vi "Run.vi"(8 "error in (no error)":errorcluster, 10 "OTP Cluster Out":T1, 11 "Measurements in":refnum<class "Measurement.lvclass">) -> (0 "error out":errorcluster, 1 "Parameters":cluster{"Name":string, "Value":string}[](array[cluster]), 2 "Canceled":bool, 3 "Measurements out":refnum<class "Measurement.lvclass">)   [LabVIEW 2020, in "Measurement.lvclass"]
doc: "This is the main test vi. It is here that the test is implemented."
uses:
  Measurement.lvclass
  Controls/OTP_Cluster.ctl
  Controls/Run States.ctl
  Devices/Controls/Change setting mode enum.ctl
  Measurement.lvclass/Measurement.ctl
  Support VI/Update parameters (array).vi
  Devices/Device.lvclass
  Devices/PIC-device/PIC-Device.lvclass
  Instruments/Power Supply/Power Supply.lvclass
  Instruments/Digital Multimeter/Digital Multimeter.lvclass
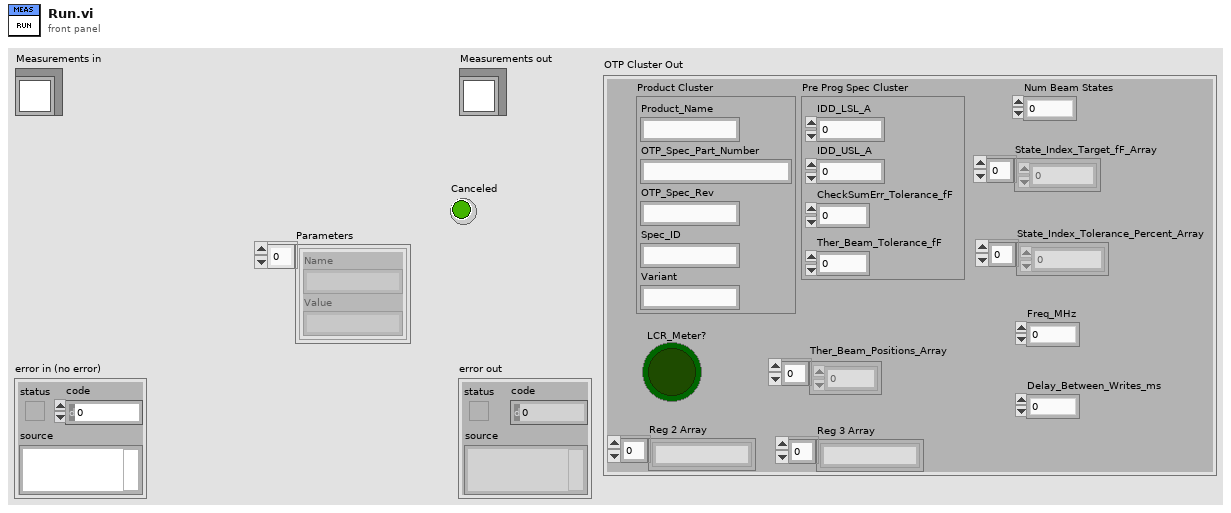
[diagram p1: front panel]
types:
  T1 = typedef "OTP_Cluster.ctl" = cluster{"Product Cluster":cluster{"Product_Name":string, "OTP_Spec_Part_Number":string, "OTP_Spec_Rev":string, "Spec_ID":string, "Variant":string}, "Pre Prog Spec Cluster":cluster{"IDD_LSL_A":dbl, "IDD_USL_A":dbl, "CheckSumErr_Tolerance_fF":dbl, "Ther_Beam_Tolerance_fF":dbl}, "LCR_Meter?":bool, "Reg 2 Array":string[], "Reg 3 Array":string[], "Num Beam States":i32, "State_Index_Target_fF_Array":dbl[], "State_Index_Tolerance_Percent_Array":dbl[], "Freq_MHz":dbl, "Delay_Between_Writes_ms":i32, "Ther_Beam_Positions_Array":i8[]}
  T2 = typedef "Measurement.lvclass/Run States.ctl" = enum16{"Init", "Set Device", "Read Environment", "Measure", "Done"}
  T3 = typedef "PIC-Device.lvclass/Change setting mode enum.ctl" = enum16{"Init", "Next", "Reset"}
  T4 = typedef "Device.lvclass/Device Information Cluster.ctl" = cluster{"Device Info":string[][], "Default Values":T5[], "Fetched info":string[][]}
  T5 = typedef "PIC-Device.lvclass/Register to Write.ctl" = cluster{"Register":u32, "Value":u32, "Dev Address":u32, "Physical Adress":u32}
  T6 = typedef "XML Handler.lvclass/Result Cluster.ctl" = cluster{"Name":string, "Value":string}
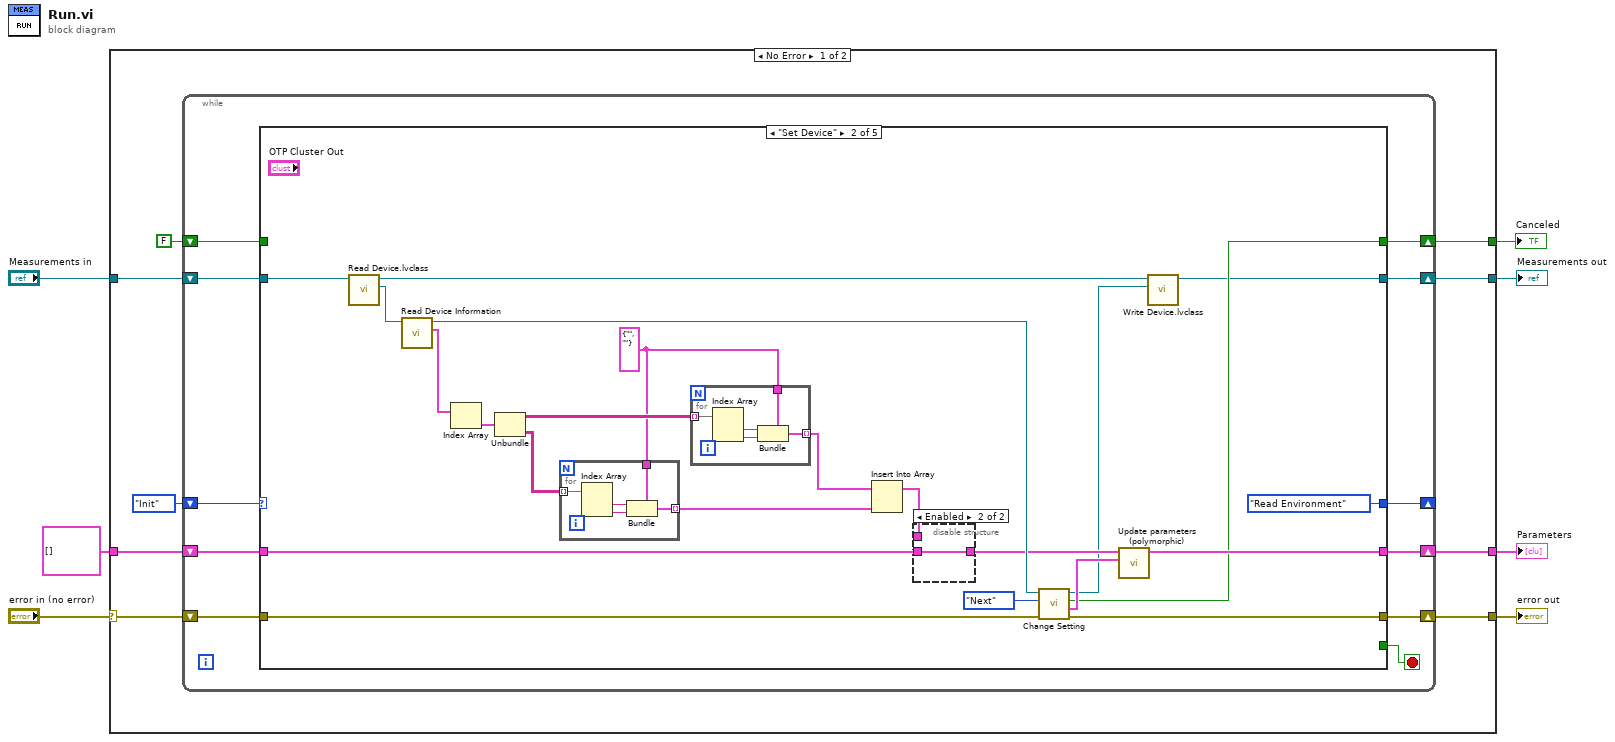
[diagram p0: block diagram]
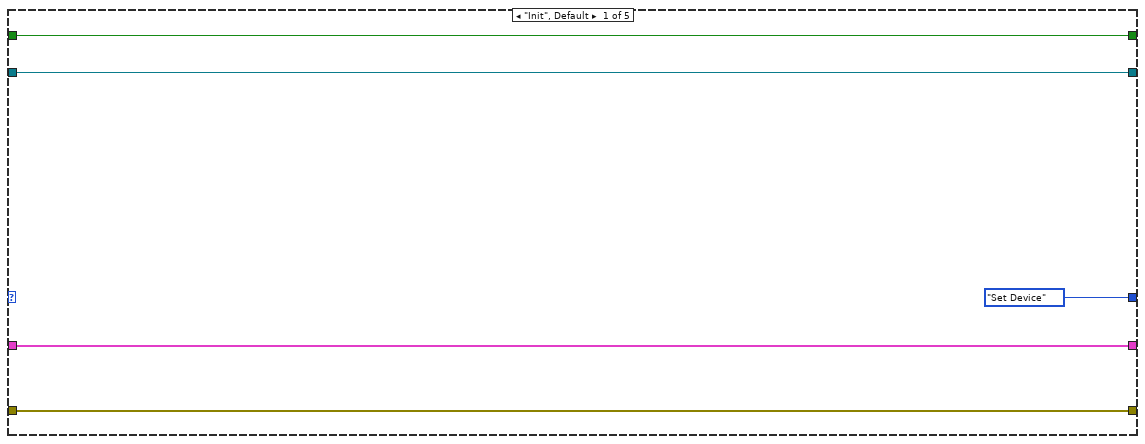
[diagram p2: hidden frame]
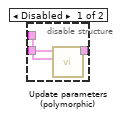
[diagram p3: hidden frame]
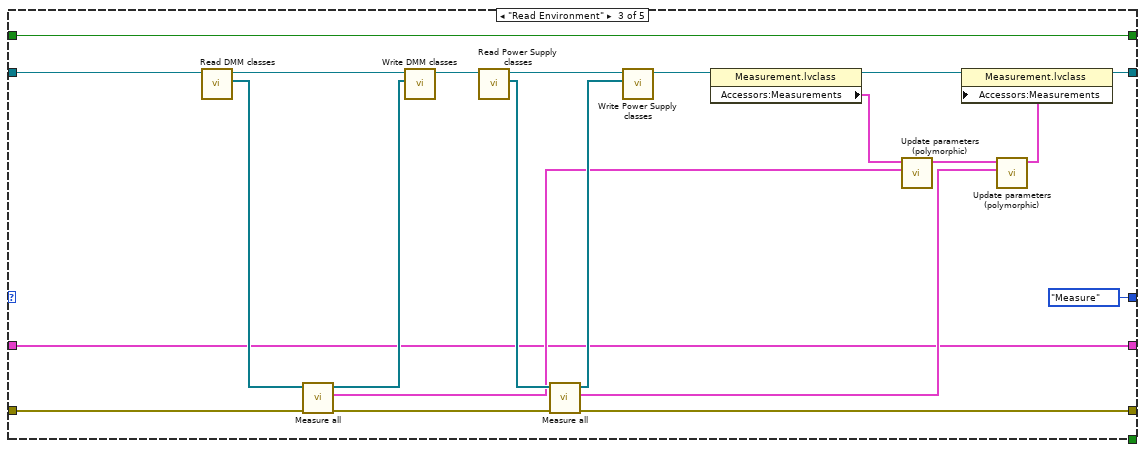
[diagram p4: hidden frame]
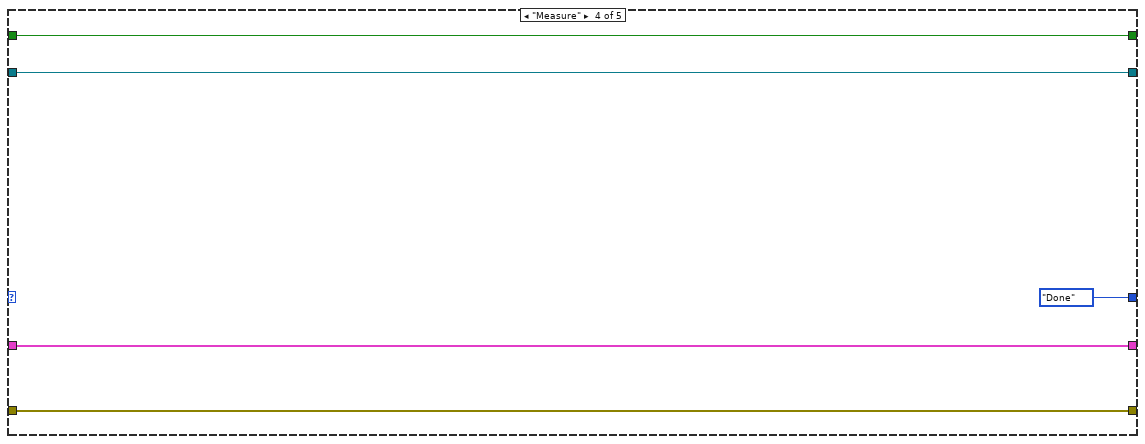
[diagram p5: hidden frame]
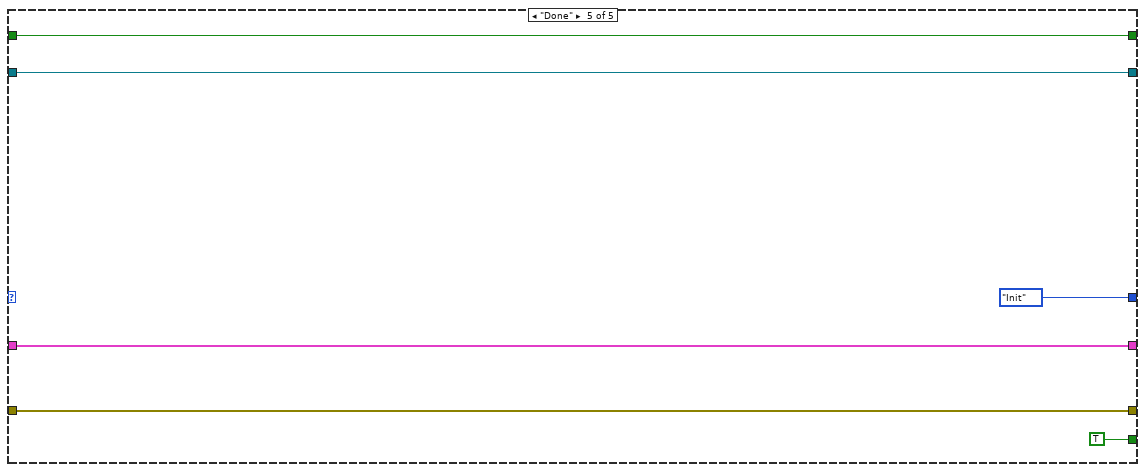
[diagram p6: hidden frame]
diagram:
  n1 = case shown="No Error" "error in (no error)" {
    selector: "error in (no error)" -> [w11 w105]
    tunnel: [w10 w105] -> w6
    tunnel: [w14 w104] -> w4
    tunnel: "Measurements in" -> [w13 w104]
    tunnel: cluster{"Name":string, "Value":string}[] [] ("Parameters") -> [w12 w103]
    tunnel: [w9 w103] -> w3
    tunnel: [w8 _] -> w1
    frame No Error {
      n2 = while {
        shift-right: [w25] -> _
        shift-left: Run_States."Init" -> [w27]
        shift-right: [w23] -> w10
        shift-left: w11 -> [w24]
        shift-right: [w22] -> w14
        shift-left: w13 -> [w26]
        shift-right: [w19] -> w9
        shift-left: w12 -> [w20]
        shift-right: [w18] -> w8
        shift-left: FALSE -> [w17]
        stop <- w21 stop-if-true
        n3 = case shown="\"Set Device\"" w27 {
          tunnel: w26 -> [w32 w49 w88 w95 w102]
          tunnel: [Run_States."Set Device" Run_States."Read Environment" Run_States."Measure" Run_States."Done" Run_States."Init"] -> w25
          tunnel: w24 -> [w28 w51 w80 w93 w101]
          tunnel: [w28 w52 w84 w93 w101] -> w23
          tunnel: [w32 w36 w71 w95 w102] -> w22
          tunnel: [_ _ _ _ TRUE] -> w21
          tunnel: w20 -> [w31 w44 w70 w94 w99]
          tunnel: [w31 w50 w70 w94 w99] -> w19
          tunnel: [w29 w48 w90 w92 w97] -> w18
          tunnel: w17 -> [w29 _ w90 w92 w97]
          frame "Init", Default {
          }
          frame "Set Device" {
            w33 = cluster{"Name":string, "Value":string} {"Name"="", "Value"=""} ("New Parameter")
            n4 = call "Read Device.lvclass.vi"("Measurements in"=w49) -> ("Device.lvclass"=w47:refnum<class "Device.lvclass">, "Measurements out"=w37:refnum<class "Measurement.lvclass">)  [unwired: 9 in]
            n5 = call-dynamic "Read Device Information.vi"("Device in"=w47) -> ("Device Info"=w43:T4[], "Device out"=w46:refnum<class "Device.lvclass">)  [unwired: 8 in, 1 out]
            n6 = Index Array(array=w43) -> (element=w42:T4)  [unwired: 1 in]
            n7 = Unbundle(w42) -> ("Device Info"=w39:string[][], "Fetched info"=w35:string[][])  [unwired: 1 out]
            n8 = for {
              tunnel: w33 -> [w60]
              tunnel: [w56] -> w34 mode=indexing
              tunnel: w35 -> [w59] mode=indexing
              n9 = Index Array(array=w59) -> (element #1=w58:string, element #2=w57:string)  [unwired: 2 in]
              n10 = Bundle(cluster=w60, "Name"=w58, "Value"=w57) -> (w56:cluster{"Name":string, "Value":string})
            }
            n11 = for {
              tunnel: w33 -> [w69]
              tunnel: [w65] -> w41 mode=indexing
              tunnel: w39 -> [w68] mode=indexing
              n12 = Index Array(array=w68) -> (element #1=w67:string, element #2=w66:string)  [unwired: 2 in]
              n13 = Bundle(cluster=w69, "Name"=w67, "Value"=w66) -> (w65:cluster{"Name":string, "Value":string})
            }
            n14 = Insert Into Array(array=w41, new element=w34) -> (w40:cluster{"Name":string, "Value":string}[])  [unwired: 1 in]
            n15 = disable-structure shown="Enabled" {
              disable-tunnel: [w63 w64] -> w45
              disable-tunnel: w44 -> [w62 w64]
              disable-tunnel: w40 -> [w61 _]
              frame Disabled {
                n16 = call-poly "Update parameters (polymorphic).vi"("New Parameters"=w61, "Parameters"=w62) -> ("Parameters Out"=w63:cluster{"Name":string, "Value":string}[])  [unwired: 9 in]
              }
              frame Enabled {
              }
            }
            n17 = call-dynamic "Change Setting.vi"("error in (no error)"=w51, "Change setting mode"=Change_setting_mode_enum."Next", "Device in"=w46) -> ("error out"=w52:errorcluster, "Changes"=w53:cluster{"Name":string, "Value":string}[], "Last setting"=w48:bool, "Device out"=w38:refnum<class "Device.lvclass">)  [unwired: 5 in]
            n18 = call-poly "Update parameters (polymorphic).vi"("New Parameters"=w53, "Parameters"=w45) -> ("Parameters Out"=w50:cluster{"Name":string, "Value":string}[])  [unwired: 9 in]
            n19 = call "Write Device.lvclass.vi"("Device.lvclass"=w38, "Measurements in"=w37) -> ("Measurements out"=w36:refnum<class "Measurement.lvclass">)  [unwired: 9 in]
          }
          frame "Read Environment" {
            n20 = call-dynamic "Read DMM classes.vi"("Measurements in"=w88) -> ("DMM classes"=w82:refnum<class "Digital Multimeter.lvclass">[], "Measurements out"=w89:refnum<class "Measurement.lvclass">)  [unwired: 9 in]
            n21 = call "Measure all.vi"("error in (no error)"=w80, "Digital Multimeters in"=w82) -> ("error out"=w79:errorcluster, "Measurements"=w77:T6[], "Digital Multimeters out"=w81:refnum<class "Digital Multimeter.lvclass">[])  [unwired: 5 in, 2 out]
            n22 = call-dynamic "Write DMM classes.vi"("DMM classes"=w81, "Measurements in"=w89) -> ("Measurements out"=w83:refnum<class "Measurement.lvclass">)  [unwired: 9 in]
            n23 = call-dynamic "Read Power Supply classes.vi"("Measurements in"=w83) -> ("Power Supply classes"=w86:refnum<class "Power Supply.lvclass">[], "Measurements out"=w87:refnum<class "Measurement.lvclass">)  [unwired: 9 in]
            n24 = call "Measure all.vi"("error in (no error)"=w79, "Power Supplies in"=w86) -> ("error out"=w84:errorcluster, "Measurements"=w74:T6[], "Power Supplies out"=w85:refnum<class "Power Supply.lvclass">[])  [unwired: 5 in, 2 out]
            n25 = call-dynamic "Write Power Supply classes.vi"("Power Supply classes"=w85, "Measurements in"=w87) -> ("Measurements out"=w72:refnum<class "Measurement.lvclass">)  [unwired: 9 in]
            n26 = property class="Measurement.lvclass"(reference=w72) -> (reference out=w78:refnum<class "Measurement.lvclass">, "Accessors:Measurements"=w76:cluster{"Name":string, "Value":string}[])  [unwired: 1 in, 1 out]
            n27 = call-poly "Update parameters (polymorphic).vi"("New Parameters"=w77, "Parameters"=w76) -> ("Parameters Out"=w75:cluster{"Name":string, "Value":string}[])  [unwired: 9 in]
            n28 = call-poly "Update parameters (polymorphic).vi"("New Parameters"=w74, "Parameters"=w75) -> ("Parameters Out"=w73:cluster{"Name":string, "Value":string}[])  [unwired: 9 in]
            n29 = property class="Measurement.lvclass"(reference=w78, "Accessors:Measurements"=w73) -> (reference out=w71:refnum<class "Measurement.lvclass">)  [unwired: 1 in, 1 out]
          }
          frame "Measure" {
          }
          frame "Done" {
          }
        }
      }
    }
    frame Error {
    }
  }
  "error out" <- w6
  "Measurements out" <- w4
  "Canceled" <- w1
  "Parameters" <- w3
